vi "Creat File With Autocreate Folder.vi"(6 "source path":path, 8 "error in (no error)":errorcluster, 10 "File Base Path":path, 11 "File Path":path) -> (0 "error out":errorcluster, 2 "New File(False)":bool, 3 "File Path Out":path)   [LabVIEW 2015]
uses:
  <vilib>/Utility/error.llb/Error Cluster From Error Code.vi
  <vilib>/ErrorRing/Error Ring.xnode
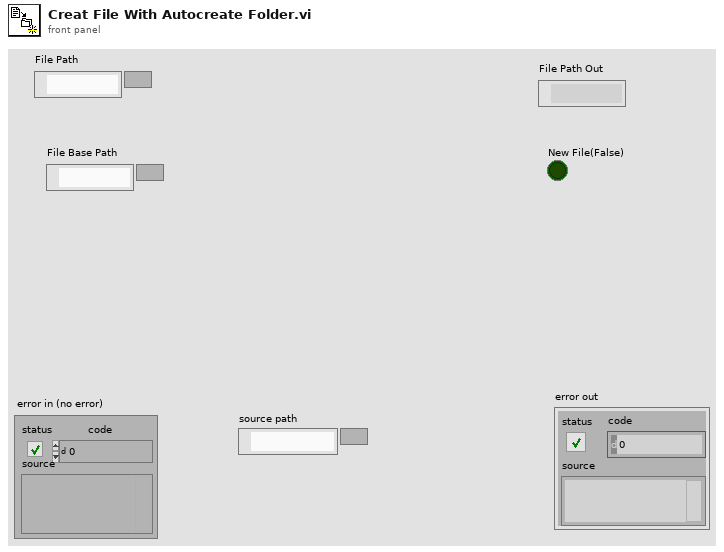
[diagram p1: front panel]
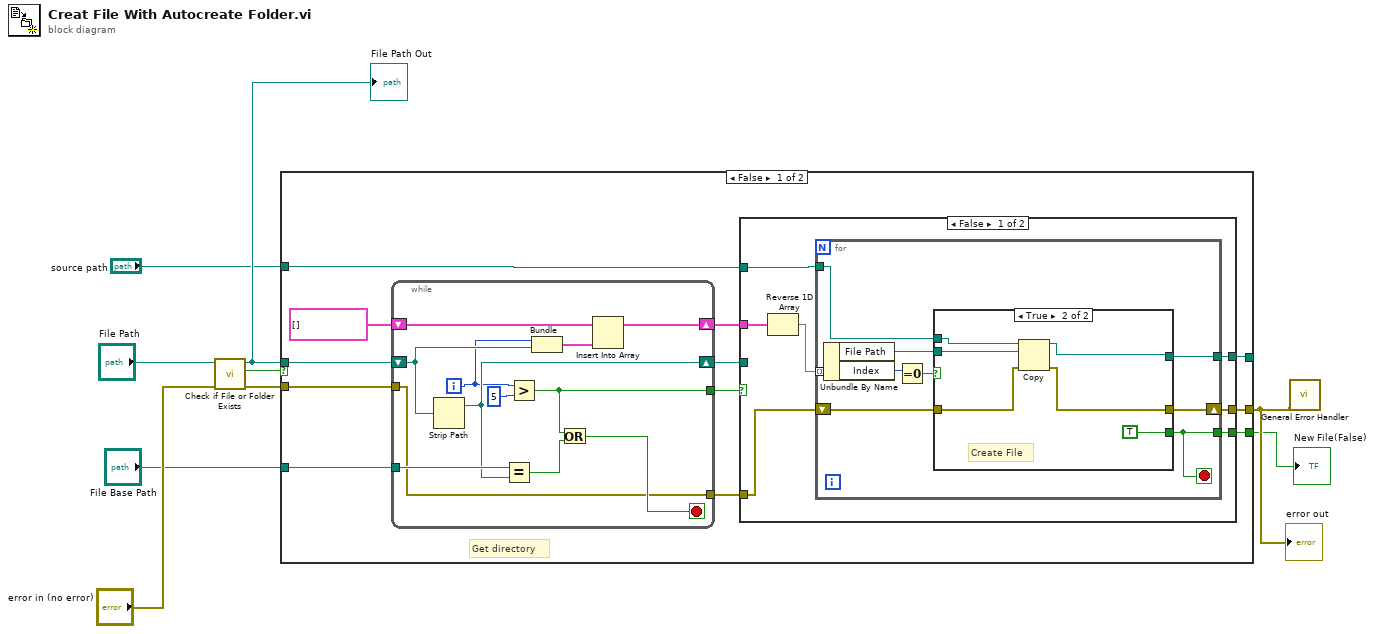
[diagram p0: block diagram]
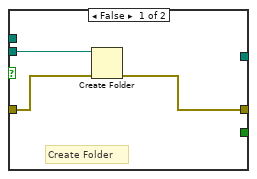
[diagram p2: hidden frame]
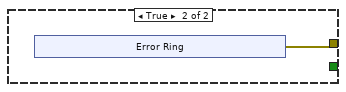
[diagram p3: hidden frame]
diagram:
  n1 = call <vilib>:"Check if File or Folder Exists.vi"("error in (no error)"="error in (no error)", "path"="File Path") -> ("error out"=w6:errorcluster, "file or folder exists?"=w7:bool, "dup path"=w2:path)  [unwired: 7 in]
  "File Path Out" <- w2
  n2 = case shown="False" w7 {
    tunnel: w6 -> [w20 w65]
    tunnel: w2 -> [w21 _]
    tunnel: "File Base Path" -> [w19 _]
    tunnel: [w13 w65] -> w4
    tunnel: [w12 _] -> w3
    tunnel: [w11 _] -> _
    tunnel: "source path" -> [w10 _]
    frame False {
      # "Get directory"
      n3 = while {
        tunnel: w20 -> [w53]
        tunnel: w19 -> [w64]
        shift-right: [w60] -> w16
        shift-left: cluster{"Index":i32, "File Path":path}[] [] -> [w62]
        shift-right: [w59] -> w15
        shift-left: w21 -> [w63]
        tunnel: [w54] -> w17
        tunnel: [w53] -> w14
        i -> [w58]
        stop <- w55 stop-if-true
        n4 = Strip Path(path=w63) -> (stripped path=w59:path)  [unwired: 1 out]
        n5 = Equal?(x=w64, y=w59) -> (x = y?=w56:bool)
        n6 = Greater?(x=w58, y=5) -> (0:w54:bool)
        n7 = Bundle(w58, "dup path"=w63) -> (w61:cluster{i32, "dup path":path})  [unwired: 1 in]
        n8 = Or(x=w54, y=w56) -> (x .or. y?=w55:bool)
        n9 = Insert Into Array(array=w62, new element=w61) -> (w60:cluster{"Index":i32, "File Path":path}[])  [unwired: 1 in]
      }
      n10 = case shown="False" w17 {
        tunnel: w16 -> [w28 _]
        tunnel: w15 -> [_ _]
        tunnel: w14 -> [w26 _]
        tunnel: [w25 w47] -> w13
        tunnel: [w24 _] -> w12
        tunnel: [w23 _] -> w11
        tunnel: w10 -> [w22 _]
        frame False {
          n11 = Reverse 1D Array(array=w28) -> (reversed array=w27:cluster{"Index":i32, "File Path":path}[])
          n12 = for {
            tunnel: w27 -> [w37] mode=indexing
            shift-right: [w32] -> w25
            shift-left: w26 -> [w33]
            tunnel: [w31] -> w24
            tunnel: [w30] -> w23
            tunnel: w22 -> [w29]
            stop <- w31 stop-if-true
            n13 = Unbundle By Name(w37) -> ("File Path"=w34:path, "Index"=w36:i32)
            n14 = Equal To 0?(x=w36) -> (x = 0?=w35:bool)
            n15 = case shown="True" w35 {
              tunnel: w34 -> [w40 w45]
              tunnel: w33 -> [w39 w43]
              tunnel: [w38 w41] -> w32
              tunnel: [_ TRUE] -> w31
              tunnel: [_ w42] -> w30
              tunnel: w29 -> [_ w44]
              frame False {
                # "Create Folder"
                n16 = Create Folder(path (use dialog)=w40, error in=w39) -> (error out=w38:errorcluster)  [unwired: 1 in, 2 out]
              }
              frame True {
                # "Create File"
                n17 = Copy(8:w43, 10:w45, 11:w44) -> (0:w41:errorcluster, 3:w42:path)  [unwired: 2 in, 1 out]
              }
            }
          }
        }
        frame True {
          n18 = xnode "Error Ring"() -> ("error out"=w47:errorcluster)
        }
      }
    }
    frame True {
    }
  }
  "error out" <- w4
  "New File(False)" <- w3
  n19 = call <vilib>:"General Error Handler.vi"("error in (no error)"=w4) -> ()  [unwired: 10 in, 5 out]
